vi "Analyser Reset.vi"(6 "Analysator":T2="N2", 8 "error in (no error)":errorcluster caption="Fehler (Eingang, kein Fehler)", 11 "Kombinationsfeld (Eingang)":refnum<vi>) -> (0 "error out":errorcluster caption="Fehler (Ausgang)", 3 "Strings und Werte []":T1)   [LabVIEW 2020, in "System Einstellungen V2.lvlib"]
uses:
  System Einstellungen V2.lvlib
  Analysatoren.ctl
  <vilib>/Utility/miscctls.llb/LVComboBoxStrsAndValuesArrayTypeDef.ctl
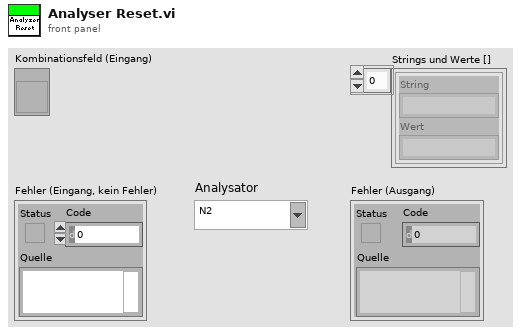
[diagram p1: front panel]
types:
  T1 = typedef "LVComboBoxStrsAndValuesArrayTypeDef.ctl" = cluster{"String":string, "Value":string}[]
  T2 = typedef "System Einstellungen V2.lvlib/Analysatoren.ctl" = string
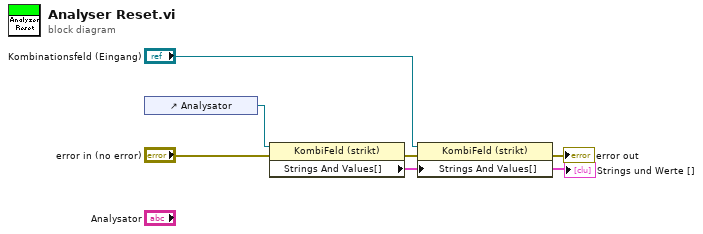
[diagram p0: block diagram]
diagram:
  n1 = control-ref of="Analysator"() -> (w6:refnum<vi>)
  n2 = property class="KombiFeld (strikt)"(reference=w6, error in="error in (no error)") -> (error out=w3:errorcluster, "Strings And Values[]"=w4:T1)  [unwired: 1 out]
  "Strings und Werte []" <- w4
  n3 = property class="KombiFeld (strikt)"(reference="Kombinationsfeld (Eingang)", error in=w3, "Strings And Values[]"=w4) -> (error out=→"error out":errorcluster)  [unwired: 1 out]
